vi "Autonomous Independent.vi"() -> ()   [LabVIEW 2014]
doc: "This VI is called when autonomous begins, and will automatically be terminated when autonomous ends. You can carry out timed or sensor driven robot movement independently without needing to return to the caller."
uses:
  <vilib>/Rock Robotics/WPI/Solenoid/Deprecated/WPI_SolenoidSetBool.vi
  <vilib>/Rock Robotics/Network Tables/SD Write Number.vi
  <vilib>/Rock Robotics/Network Tables/SD Read Number.vi
panel:
  out "JDF Distance":dbl
  out "JDF Speed":dbl
  out "Speed 2":dbl
  out "Speed 1":dbl
  out "Placing Distance":dbl
  out "Turning Angle":dbl
  out "Distance 2":dbl
  out "Distance 1":dbl
  in  "Reset Encoder":bool
  in  "3 Tote Data":T1
  out "Pot Value":dbl
  out "Avg Encoder":dbl
  out "R Encoder":dbl
  out "L Encoder":dbl
  # "3.5\n1.5\n80\n8\n.6\n.7"
  # "85\n4.5"
  # "Be sure to right-click and choose Data Operations>>Make Current Value default if you want to save the array values with the VI"
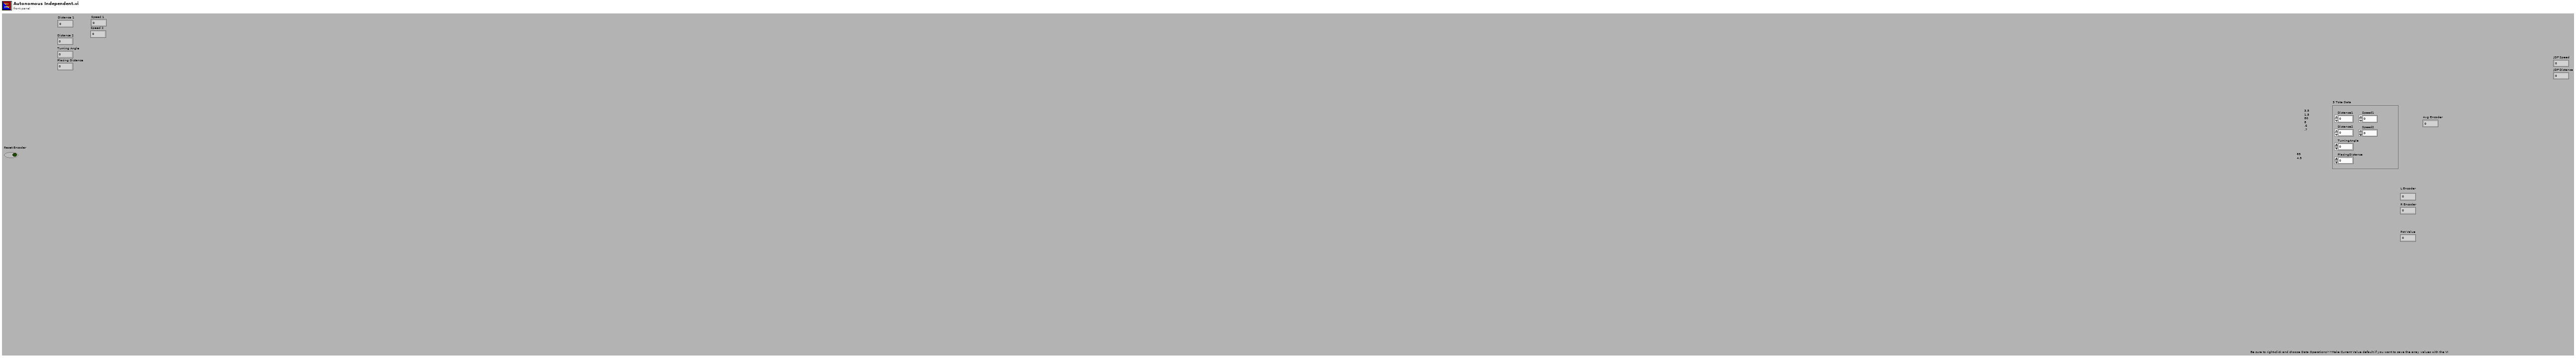
[diagram p1: front panel]
types:
  T1 = cluster{"Distance1":dbl, "Distance2":dbl, "TurningAngle":dbl, "PlacingDistance":dbl, "Speed1":dbl, "Speed2":dbl}
  T2 = typedef "WPI_SolenoidDevRef.ctl" = cluster{"DevStatus":errorcluster, "Pneumatics Control Module":u8, "Forward Solenoid Channel":T3, "Reverse Solenoid Channel":T3}
  T3 = typedef "WPI_SolenoidChannel.ctl" = enum8{"Solenoid 0", "Solenoid 1", "Solenoid 2", "Solenoid 3", "Solenoid 4", "Solenoid 5", "Solenoid 6", "Solenoid 7", "Invalid"}
  T4 = typedef "WPI_MotorControlDeviceRef.ctl" = cluster{"DeviceStatus":errorcluster, "Type":T5, "PWM":cluster{"Controller":T6, "PWM Channel":T7, "DeadBand":T8}, "CAN":cluster{"Device Number":u8, "Control Mode":T9, "Semaphore":T10, "Max Vout":dbl, "TalonSRX Control Mode":T11}, "Invert":bool, "TransformRef":T12, "InvTransformRef":T12}
  T5 = typedef "WPI_MotorControlType.ctl" = enum16{"PWM", "CAN", "CANTalonSRX"}
  T6 = typedef "FPGA_TypedefDigitalModule.ctl" = enum16{"Controller 1"}
  T7 = typedef "FPGA_DIOPWMChannel.ctl" = enum8{"PWM 0", "PWM 1", "PWM 2", "PWM 3", "PWM 4", "PWM 5", "PWM 6", "PWM 7", "PWM 8", "PWM 9", "PWM MXP 0", "PWM MXP 1", "PWM MXP 2", "PWM MXP 3", "PWM MXP 4", "PWM MXP 5", "PWM MXP 6", "PWM MXP 7", "PWM MXP 8", "PWM MXP 9", "Invalid"}
  T8 = typedef "WPI_PWMDeadband.ctl" = cluster{"Name":string, "maxPositivePwm":i32, "minPositivePwm":i32, "centerPwm":i32, "maxNegativePwm":i32, "minNegativePwm":i32, "angularRange":u16}
  T9 = typedef "WPI_CANJaguar_ControlMode.ctl" = enum8{"Percent VBus", "Current", "Speed", "Position", "Voltage"}
  T10 = typedef "Semaphore RefNum" = refnum<k1>
  T11 = typedef "WPI_CANTalonSRX_APIControlMode.ctl" = enum8{"Percent VBus", "Speed", "Position", "Slave", "Unchanged / Invalid"}
  T12 = typedef "WPI_PWMTransform_ConPane.ctl" = refnum<vi>
  T13 = typedef "WPI_RobotDriveDevRef.ctl" = cluster{"DevStatus":errorcluster, "Motors[]":T4[], "Square Inputs":bool, "Max Output":dbl}
  T14 = cluster{"SolenoidDevRef":T2, "SolenoidDevRef":T2, "MotorControlDevRef":T4, "MotorControlDevRef":T4, "SolenoidDevRef":T2, "SolenoidDevRef":T2, "SolenoidDevRef":T2}
  T15 = cluster{"SolenoidDevRef":T2, "SolenoidDevRef":T2, "MotorControlDevRef":T4, "RobotDriveDevRef":T13}
  T16 = typedef "WPI_GyroDevRef.ctl" = cluster{"DevStatus":errorcluster, "Analog Module":T17, "Analog Channel":T18, "Offset":dbl, "Gain (VoltsPerDegree/Second)":dbl}
  T17 = typedef "FPGA_TypedefAnalogModule.ctl" = enum16{"Controller 1"}
  T18 = typedef "FPGA_AIChannel.ctl" = enum8{"AI 0", "AI 1", "AI 2", "AI 3", "AI MXP 0", "AI MXP 1", "AI MXP 2", "AI MXP 3", "Invalid"}
  T19 = typedef "WPI_PotentiometerDevRef.ctl" = cluster{"DevStatus":errorcluster, "Controller":T17, "Analog Channel":T18, "Invert Output":bool}
  T20 = typedef "WPI_EncoderDevRef.ctl" = cluster{"DevStatus":errorcluster, "EncoderIndex":T21, "CounterIndex":T22, "DistancePerCount":dbl, "Decoding Type":T23}
  T21 = typedef "FPGA_EncoderIdx.ctl" = enum8{"Enc 0", "Enc 1", "Enc 2", "Enc 3", "Enc 4", "Enc 5", "Enc 6", "Enc 7", "Invalid"}
  T22 = typedef "FPGA_CounterCtrSystemIndex.ctl" = enum8{"Ctr 0", "Ctr 1", "Ctr 2", "Ctr 3", "Ctr 4", "Ctr 5", "Ctr 6", "Ctr 7", "Invalid"}
  T23 = typedef "WPI_EncoderType.ctl" = enum16{"1x", "2x", "4x"}
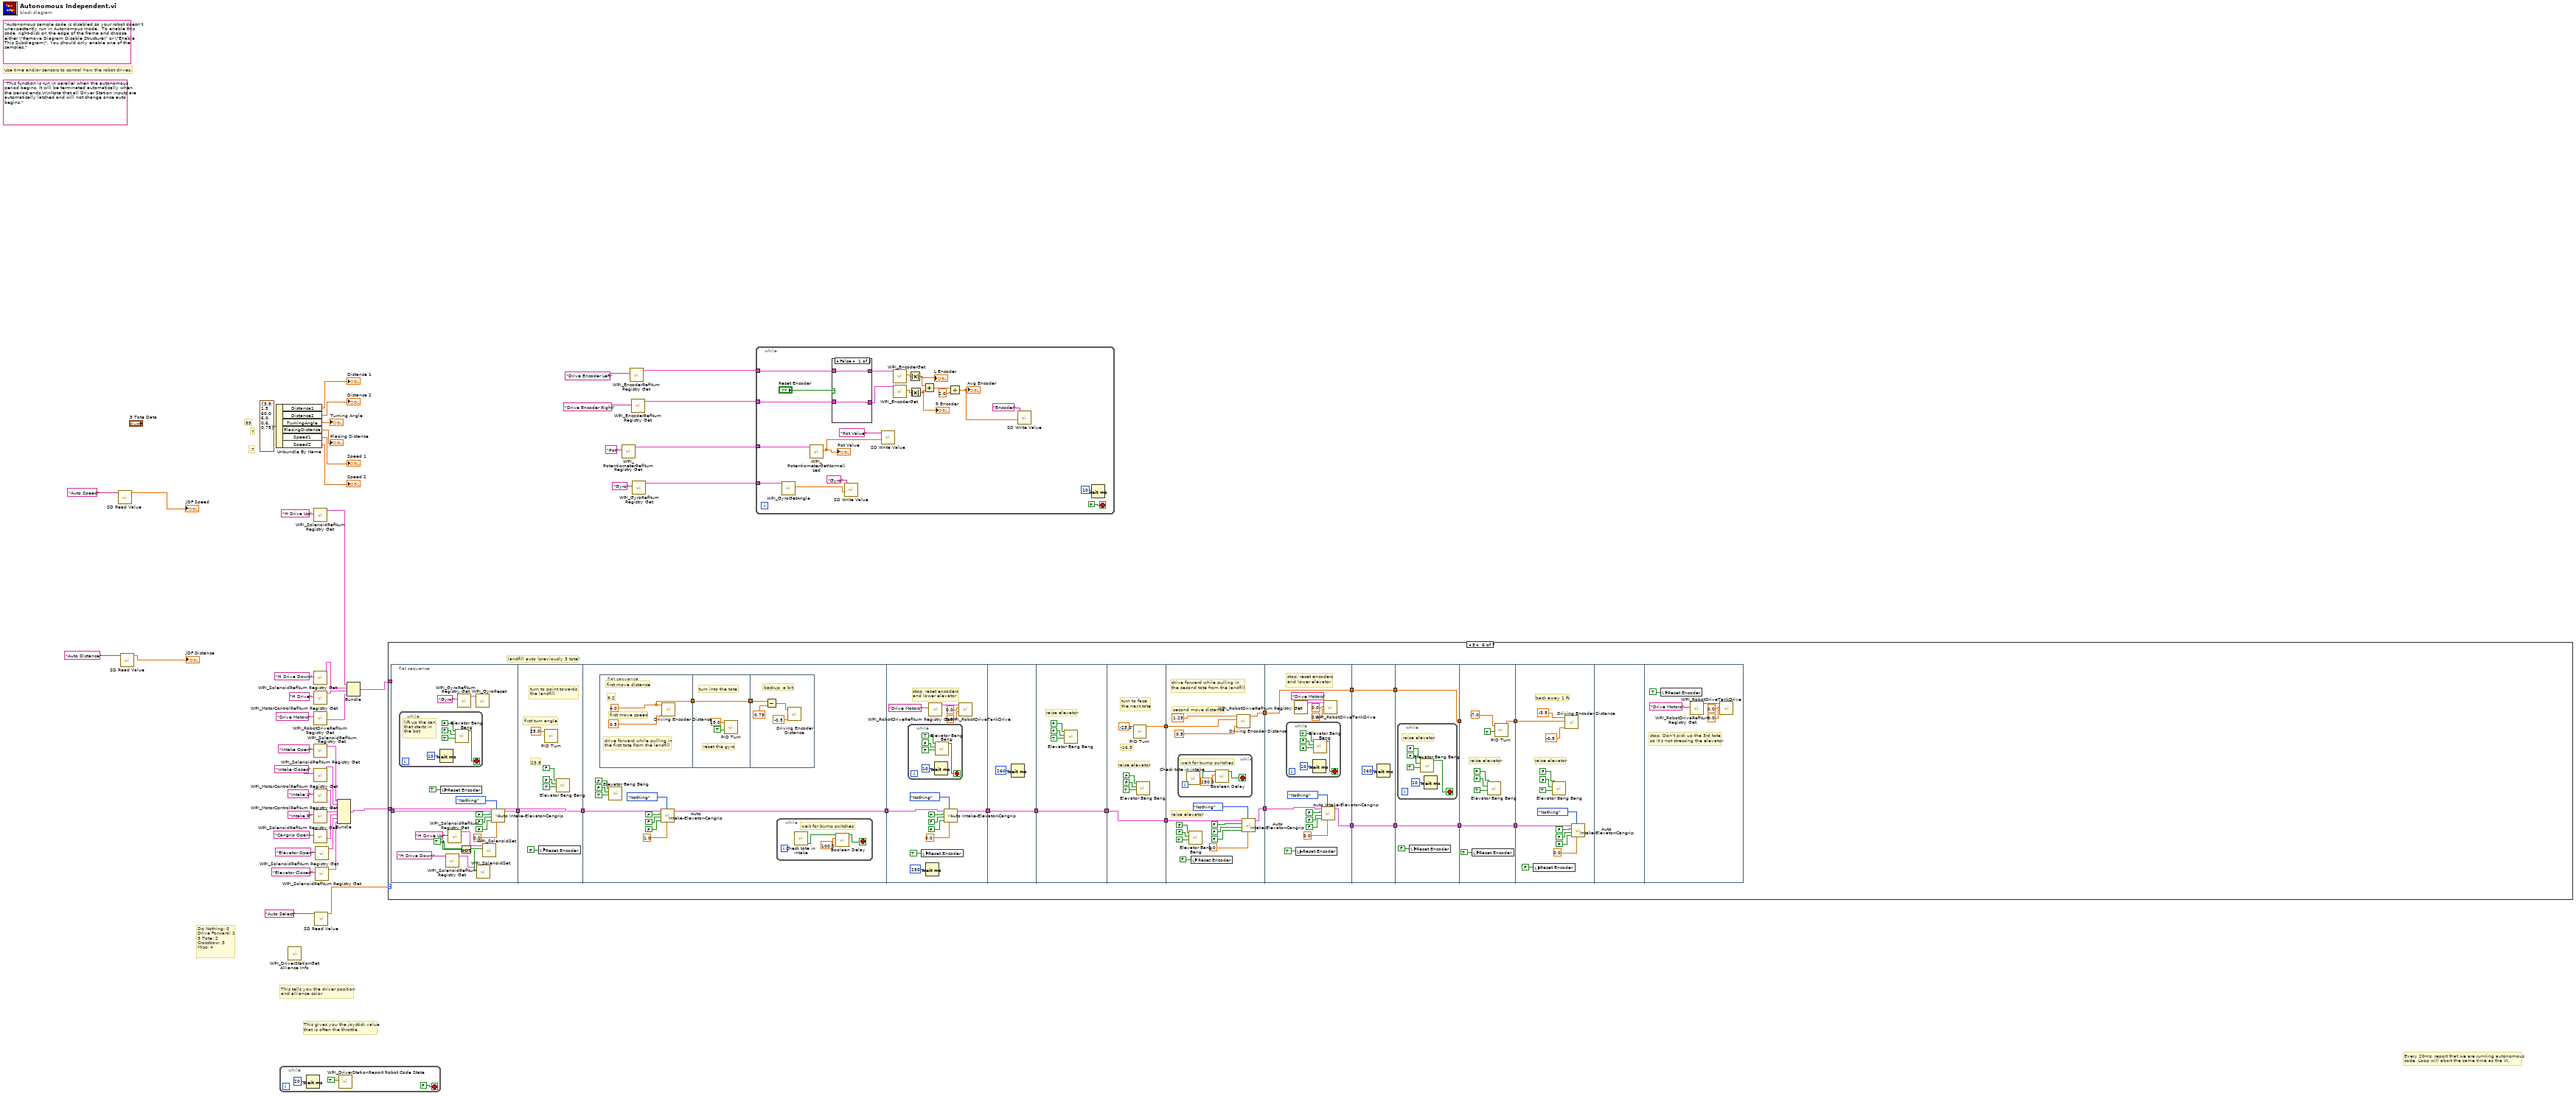
[diagram p0: block diagram]
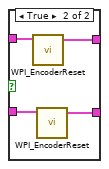
[diagram p2: hidden frame]
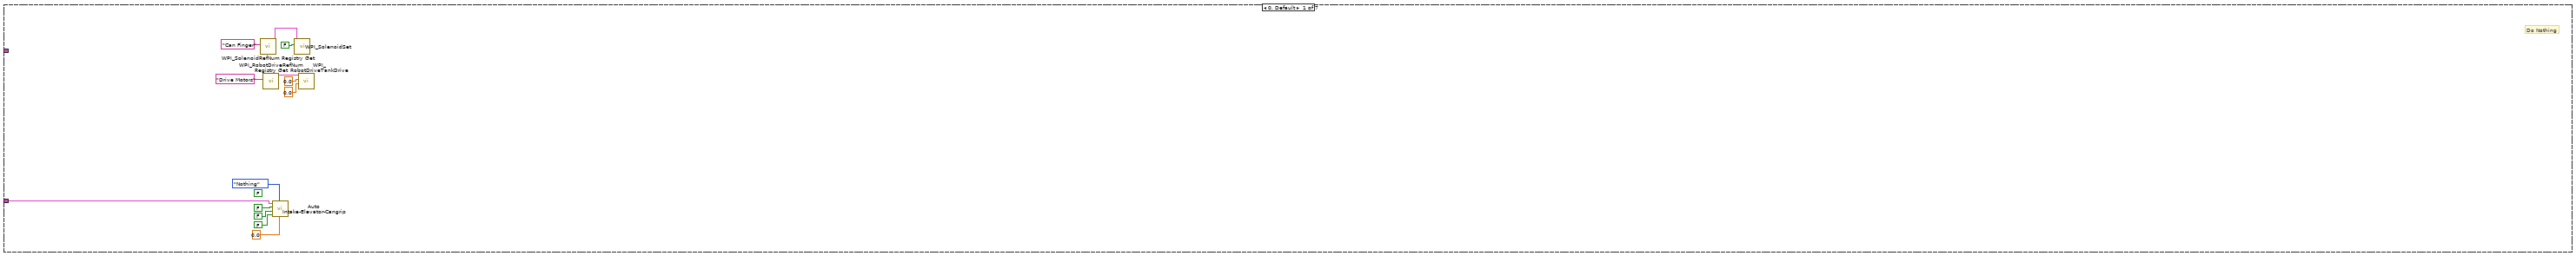
[diagram p3: hidden frame]
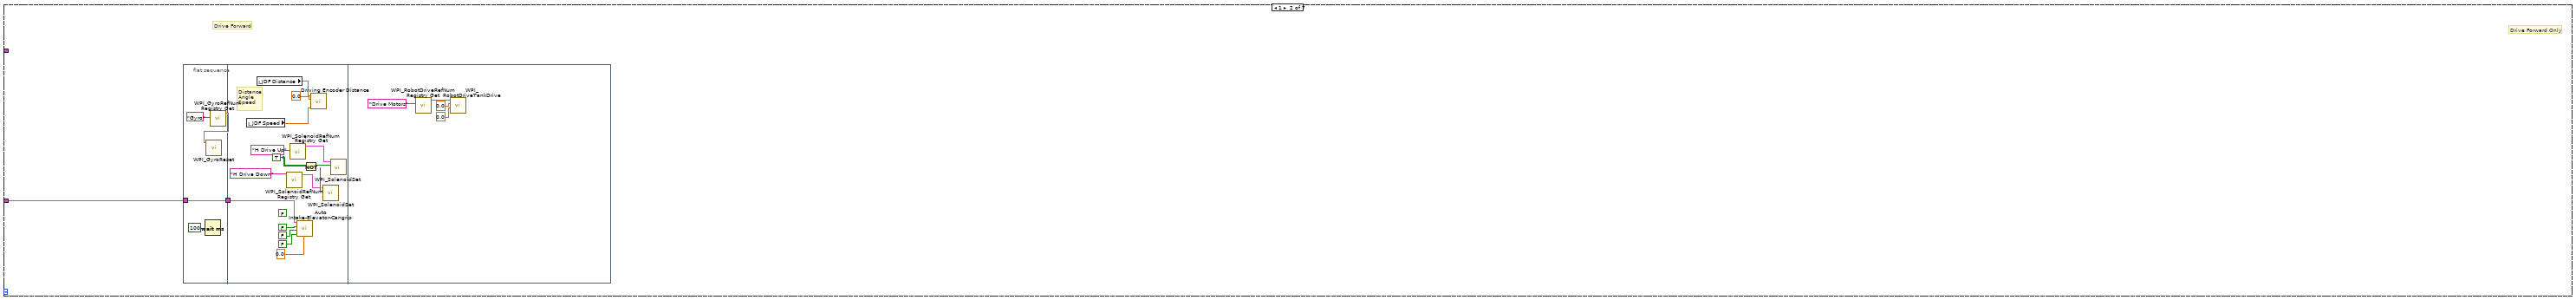
[diagram p4: hidden frame]
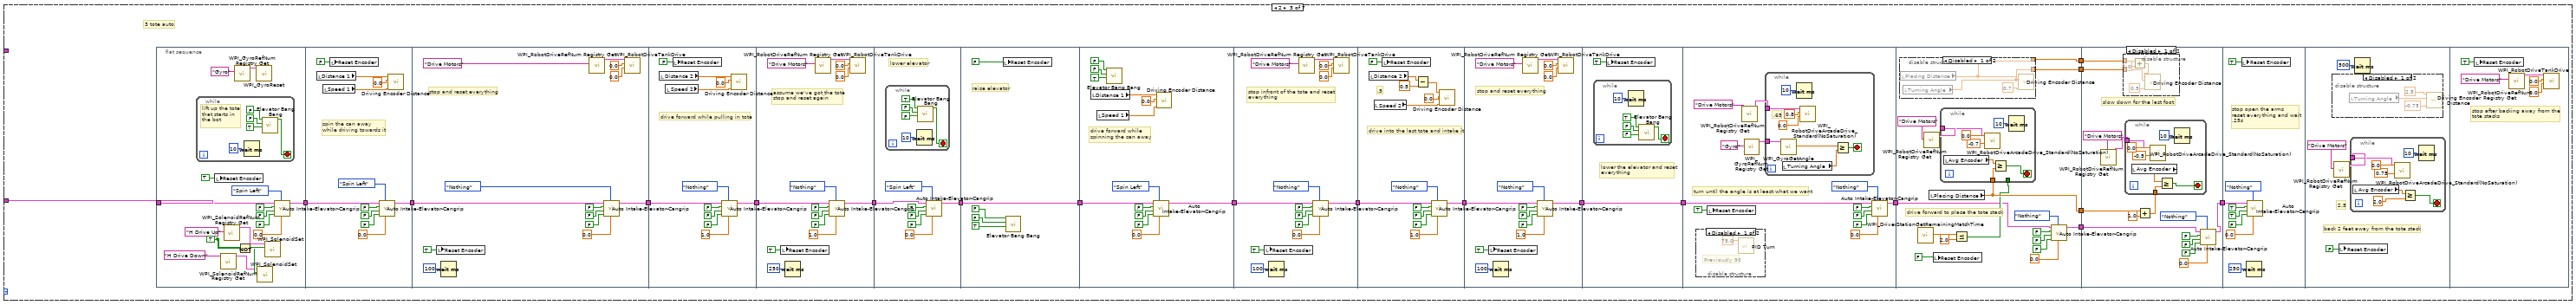
[diagram p5: hidden frame]
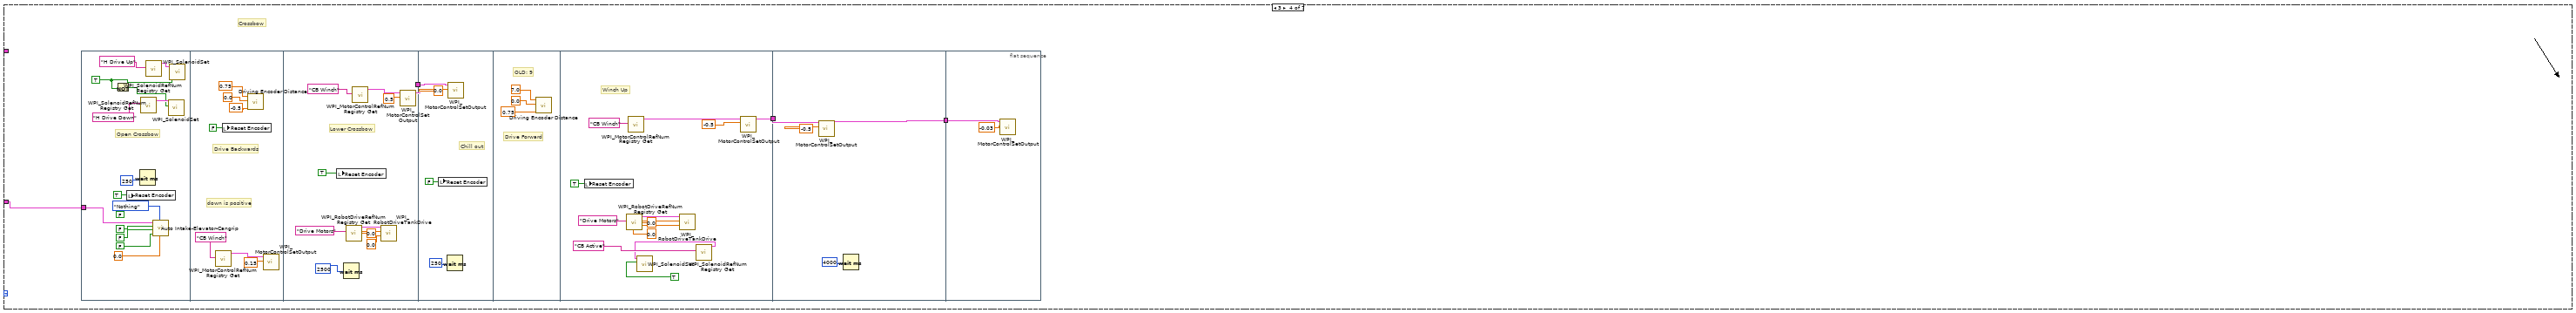
[diagram p10: hidden frame]
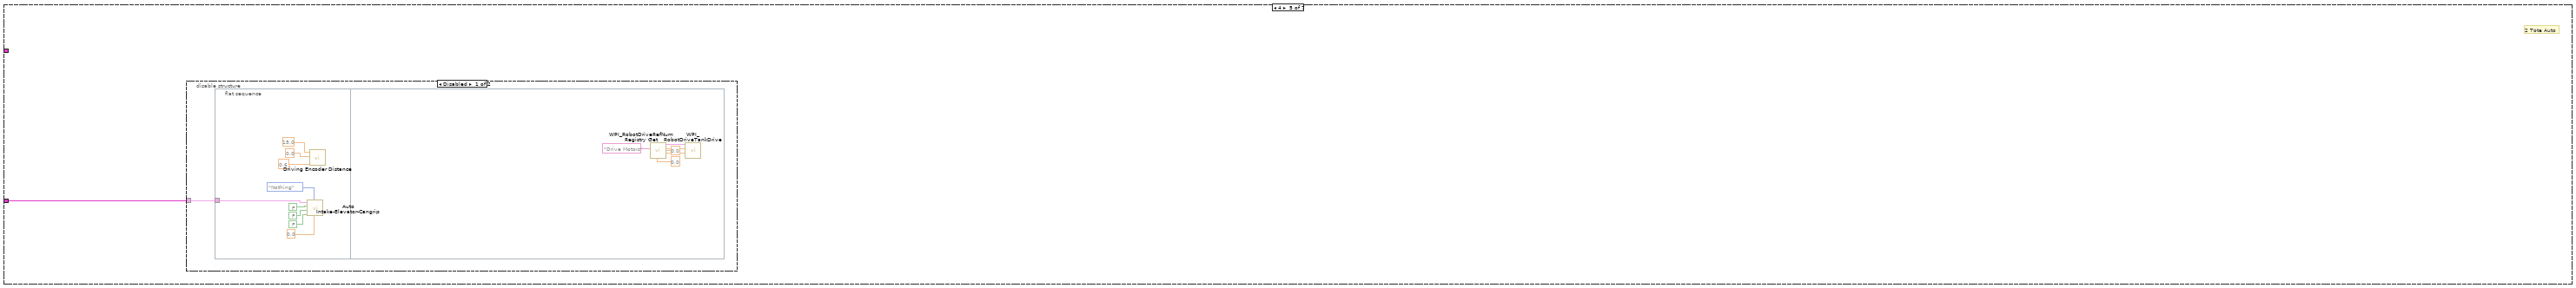
[diagram p11: hidden frame]
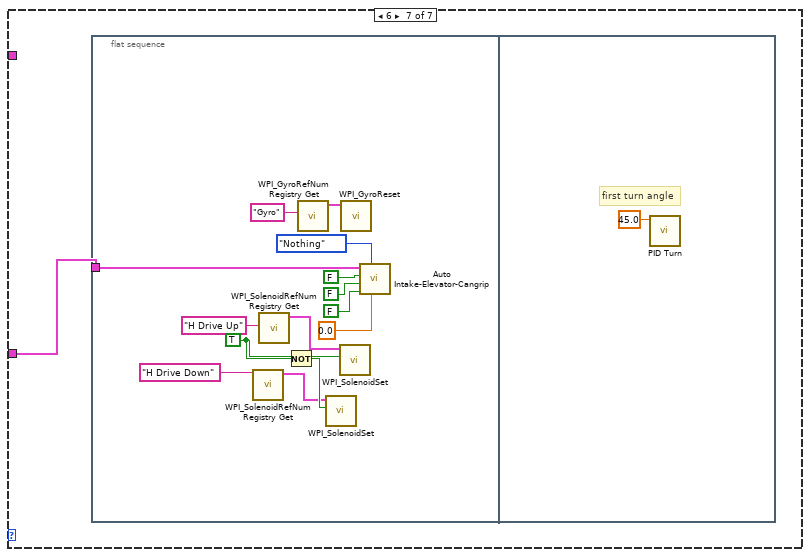
[diagram p13: hidden frame]
diagram:
  (unwired) "Autonomous sample code is disabled so your robot doesn't unexpectantly run in Autonomous mode.  To enable this code, right-click on the edge of the frame and choose either \"Remove Diagram Disable Structure\" or \"Enable This Subdiagram\". You should only enable one of the samples."
  (unwired) "This function is run in parallel when the autonomous period begins. It will be terminated automatically when the period ends.\n\nNote that all Driver Station inputs are automatically latched and will not change once auto begins."
  # "7"
  # "85"
  # ".7"
  # "Do Nothing: 0\nDrive Forward: 1\n3 Tote: 2\nCrossbow: 3\nMisc: 4"
  # "Every 20ms, report that we are running autonomous\ncode. Loop will abort the same time as the VI."
  # "This gives you the joystick value\nthat is often the throttle"
  # "Use time and/or sensors to control how the robot drives."
  # "This tells you the driver position\nand alliance color"
  n1 = call-poly <vilib>:"SD Read Value.vi"("Name"="Auto Speed") -> ("Numeric"=→"JDF Speed":dbl)  [unwired: 8 in, 2 out]
  n2 = call-poly <vilib>:"SD Read Value.vi"("Name"="Auto Distance") -> ("Numeric"=→"JDF Distance":dbl)  [unwired: 8 in, 2 out]
  n3 = Unbundle By Name(T1 {"Distance1"=3.5, "Distance2"=1.5, "TurningAngle"=60.0, "PlacingDistance"=6.0, "Speed1"=0.6, "Speed2"=0.75} ("input cluster")) -> ("Distance1"=→"Distance 1":dbl, "Distance2"=→"Distance 2":dbl, "TurningAngle"=→"Turning Angle":dbl, "PlacingDistance"=→"Placing Distance":dbl, "Speed1"=→"Speed 1":dbl, "Speed2"=→"Speed 2":dbl)
  n4 = while {
    stop <- FALSE stop-if-true
    n5 = Wait (ms)(milliseconds to wait=u32 20) -> ()  [unwired: 1 out]
    n6 = call <vilib>:"WPI_DriverStationReport Robot Code State.vi"("Autonomous"=TRUE) -> ()  [unwired: 10 in, 1 out]
  }
  n7 = call <vilib>:"WPI_DriverStationGet Alliance Info.vi"() -> ()  [unwired: 12 out]
  n8 = call <vilib>:"WPI_SolenoidRefNum Registry Get.vi"("refnum name"="H Drive Up") -> ("SolenoidDevRef"=w36:T2)  [unwired: 9 in, 1 out]
  n9 = call <vilib>:"WPI_SolenoidRefNum Registry Get.vi"("refnum name"="H Drive Down") -> ("SolenoidDevRef"=w35:T2)  [unwired: 9 in, 1 out]
  n10 = call <vilib>:"WPI_MotorControlRefNum Registry Get.vi"("refnum name"="H Drive") -> ("MotorControlDevRef"=w34:T4)  [unwired: 9 in, 1 out]
  n11 = call <vilib>:"WPI_RobotDriveRefNum Registry Get.vi"("refnum name"="Drive Motors") -> ("RobotDriveDevRef"=w33:T13)  [unwired: 1 in, 9 out]
  n12 = call <vilib>:"WPI_SolenoidRefNum Registry Get.vi"("refnum name"="Intake Open") -> ("SolenoidDevRef"=w24:T2)  [unwired: 9 in, 1 out]
  n13 = call <vilib>:"WPI_SolenoidRefNum Registry Get.vi"("refnum name"="Intake Closed") -> ("SolenoidDevRef"=w23:T2)  [unwired: 9 in, 1 out]
  n14 = call <vilib>:"WPI_MotorControlRefNum Registry Get.vi"("refnum name"="Intake L") -> ("MotorControlDevRef"=w22:T4)  [unwired: 9 in, 1 out]
  n15 = call <vilib>:"WPI_MotorControlRefNum Registry Get.vi"("refnum name"="Intake R") -> ("MotorControlDevRef"=w21:T4)  [unwired: 9 in, 1 out]
  n16 = call <vilib>:"WPI_SolenoidRefNum Registry Get.vi"("refnum name"="Cangrip Open") -> ("SolenoidDevRef"=w20:T2)  [unwired: 9 in, 1 out]
  n17 = call-poly <vilib>:"SD Read Value.vi"("Name"="Auto Select") -> ("Numeric"=w1:dbl)  [unwired: 8 in, 2 out]
  n18 = call <vilib>:"WPI_SolenoidRefNum Registry Get.vi"("refnum name"="Elevator Open") -> ("SolenoidDevRef"=w19:T2)  [unwired: 9 in, 1 out]
  n19 = call <vilib>:"WPI_SolenoidRefNum Registry Get.vi"("refnum name"="Elevator Closed") -> ("SolenoidDevRef"=w18:T2)  [unwired: 9 in, 1 out]
  n20 = Bundle("SolenoidDevRef"=w24, "SolenoidDevRef"=w23, "MotorControlDevRef"=w22, "MotorControlDevRef"=w21, "SolenoidDevRef"=w20, "SolenoidDevRef"=w19, "SolenoidDevRef"=w18) -> (w17:T14)  [unwired: 1 in]
  n21 = Bundle("SolenoidDevRef"=w36, "SolenoidDevRef"=w35, "MotorControlDevRef"=w34, "RobotDriveDevRef"=w33) -> (w32:T15)  [unwired: 1 in]
  n22 = case shown="5" w1 {
    tunnel: w32 -> [_ _ _ _ _ _ _]
    tunnel: w17 -> [w50 w63 w91 w350 w410 w443 w598]
    frame 0, Default {
      (unwired) FALSE ("Intake Spin Left")
      # "Do Nothing"
      n23 = call <vilib>:"WPI_SolenoidRefNum Registry Get.vi"("refnum name"="Can Finger") -> ("SolenoidDevRef"=w61:T2)  [unwired: 9 in, 1 out]
      n24 = call <vilib>:"WPI_RobotDriveRefNum Registry Get.vi"("refnum name"="Drive Motors") -> ("RobotDriveDevRef"=w56:T13)  [unwired: 1 in, 9 out]
      n25 = call "Auto Intake-Elevator-Cangrip.vi"("Intake Wheels (+ is in)"=0.0, "Spin Can"=enum16{"Spin Left", "Spin Right", "Nothing"}."Nothing", "Cangrip Open"=FALSE, "Elevator Open"=FALSE, "Intake Open"=FALSE, "Cluster"=w50) -> ()  [unwired: 5 in, 1 out]
      n26 = call-poly <vilib>:"WPI_SolenoidSet.vi"("Value"=FALSE, "SolenoidDevRef"=w61) -> ()  [unwired: 8 in, 2 out]
      n27 = call <vilib>:"WPI_RobotDriveTankDrive.vi"("Right axis value"=0.0, "Left axis value"=0.0, "RobotDriveDevRef"=w56) -> ()  [unwired: 6 in, 3 out]
    }
    frame 1 {
      # "Drive Forward"
      # "Drive Forward Only"
      n28 = flat-sequence {
        tunnel: w63 -> [w67]
        tunnel: [w67] -> w62
        tunnel: w62 -> [w77]
        frame #0 {
          n29 = Wait (ms)(milliseconds to wait=u32 100) -> ()  [unwired: 1 out]
          n30 = call <vilib>:"WPI_GyroRefNum Registry Get.vi"("refnum name"="Gyro") -> ("GyroDevRef"=w65:T16)  [unwired: 9 in, 1 out]
          n31 = call <vilib>:"WPI_GyroReset.vi"("GyroDevRef"=w65) -> ()  [unwired: 9 in, 2 out]
        }
        frame #1 {
          w75 = TRUE ("Reset Encoder")
          (unwired) FALSE ("Intake Spin Left")
          # "Distance\nAngle\nSpeed"
          n32 = local read "JDF Speed"() -> (w68:dbl)
          n33 = local read "JDF Distance"() -> (w69:dbl)
          n34 = call <vilib>:"WPI_SolenoidRefNum Registry Get.vi"("refnum name"="H Drive Down") -> ("SolenoidDevRef"=w73:T2)  [unwired: 9 in, 1 out]
          n35 = call <vilib>:"WPI_SolenoidRefNum Registry Get.vi"("refnum name"="H Drive Up") -> ("SolenoidDevRef"=w70:T2)  [unwired: 9 in, 1 out]
          n36 = call "Auto Intake-Elevator-Cangrip.vi"("Intake Wheels (+ is in)"=0.0, "Cangrip Open"=FALSE, "Elevator Open"=FALSE, "Intake Open"=FALSE, "Cluster"=w77) -> ()  [unwired: 6 in, 1 out]
          n37 = Not(x=w75) -> (.not. x?=w74:bool)
          n38 = call "Driving Encoder Distance.vi"("Speed"=w68, "Setpoint Angle"=0.0, "Setpoint Distance"=w69) -> ()  [unwired: 6 in, 3 out]
          n39 = call-poly <vilib>:"WPI_SolenoidSet.vi"("Value"=w74, "SolenoidDevRef"=w73) -> ()  [unwired: 8 in, 2 out]
          n40 = call-poly <vilib>:"WPI_SolenoidSet.vi"("Value"=w75, "SolenoidDevRef"=w70) -> ()  [unwired: 8 in, 2 out]
        }
        frame #2 {
          n41 = call <vilib>:"WPI_RobotDriveRefNum Registry Get.vi"("refnum name"="Drive Motors") -> ("RobotDriveDevRef"=w83:T13)  [unwired: 1 in, 9 out]
          n42 = call <vilib>:"WPI_RobotDriveTankDrive.vi"("Right axis value"=0.0, "Left axis value"=0.0, "RobotDriveDevRef"=w83) -> ()  [unwired: 6 in, 3 out]
        }
      }
    }
    frame 2 {
      # "3 tote auto"
      n43 = flat-sequence {
        tunnel: [w117] -> w104
        tunnel: w91 -> [w112]
        tunnel: [w132] -> w103
        tunnel: w104 -> [w127]
        tunnel: w103 -> [w141]
        tunnel: [w139] -> w102
        tunnel: w102 -> [w158]
        tunnel: [w154] -> w101
        tunnel: w101 -> [w169]
        tunnel: [w163] -> w100
        tunnel: [w174] -> w99
        tunnel: w100 -> [w175]
        tunnel: [w189] -> w98
        tunnel: w99 -> [w189]
        tunnel: w98 -> [w199]
        tunnel: [w198] -> w97
        tunnel: w97 -> [w207]
        tunnel: [w205] -> w96
        tunnel: w96 -> [w222]
        tunnel: [w221] -> w95
        tunnel: w95 -> [w232]
        tunnel: [w231] -> w94
        tunnel: w94 -> [w244]
        tunnel: [w244] -> w93
        tunnel: w93 -> [w257]
        tunnel: [w256] -> w92
        tunnel: w92 -> [w272]
        tunnel: [w285] -> w89
        tunnel: [w284] -> w88
        tunnel: [w281] -> w87
        tunnel: [w271] -> w86
        tunnel: [w297] -> w90
        tunnel: w89 -> [w310]
        tunnel: w88 -> [w309]
        tunnel: w87 -> [w307]
        tunnel: w86 -> [w298]
        tunnel: w90 -> [w328]
        frame #0 {
          w111 = TRUE ("Reset Encoder")
          n44 = while {
            stop <- w122 stop-if-true
            # "lift up the tote\nthat starts in \nthe bot"
            n45 = Wait (ms)(milliseconds to wait=u32 10) -> ()  [unwired: 1 out]
            n46 = call "Elevator Bang Bang.vi"("Top"=TRUE, "Middle"=FALSE, "Bottom"=FALSE) -> ("in range"=w122:bool)  [unwired: 8 in]
          }
          n47 = local write "Reset Encoder"(TRUE ("Reset Encoder")) -> ()
          n48 = call <vilib>:"WPI_SolenoidRefNum Registry Get.vi"("refnum name"="H Drive Down") -> ("SolenoidDevRef"=w107:T2)  [unwired: 9 in, 1 out]
          n49 = call <vilib>:"WPI_SolenoidRefNum Registry Get.vi"("refnum name"="H Drive Up") -> ("SolenoidDevRef"=w108:T2)  [unwired: 9 in, 1 out]
          n50 = call <vilib>:"WPI_GyroRefNum Registry Get.vi"("refnum name"="Gyro") -> ("GyroDevRef"=w119:T16)  [unwired: 9 in, 1 out]
          n51 = Not(x=w111) -> (.not. x?=w110:bool)
          n52 = call <vilib>:"WPI_GyroReset.vi"("GyroDevRef"=w119) -> ()  [unwired: 9 in, 2 out]
          n53 = call-poly <vilib>:"WPI_SolenoidSet.vi"("Value"=w110, "SolenoidDevRef"=w107) -> ()  [unwired: 8 in, 2 out]
          n54 = call-poly <vilib>:"WPI_SolenoidSet.vi"("Value"=w111, "SolenoidDevRef"=w108) -> ()  [unwired: 8 in, 2 out]
          n55 = call "Auto Intake-Elevator-Cangrip.vi"("Intake Wheels (+ is in)"=0.0, "Spin Can"=enum16{"Spin Left", "Spin Right", "Nothing"}."Spin Left", "Cangrip Open"=FALSE, "Elevator Open"=FALSE, "Intake Open"=FALSE, "Cluster"=w112) -> ("Output Cluster"=w117:T14)  [unwired: 5 in]
        }
        frame #1 {
          # "spin the can away \nwhile driving towards it"
          n56 = local read "Distance 1"() -> (w129:dbl)
          n57 = local read "Speed 1"() -> (w128:dbl)
          n58 = local write "Reset Encoder"(FALSE ("Reset Encoder")) -> ()
          n59 = call "Auto Intake-Elevator-Cangrip.vi"("Intake Wheels (+ is in)"=0.0, "Spin Can"=enum16{"Spin Left", "Spin Right", "Nothing"}."Spin Left", "Cangrip Open"=FALSE, "Elevator Open"=FALSE, "Intake Open"=FALSE, "Cluster"=w127) -> ("Output Cluster"=w132:T14)  [unwired: 5 in]
          n60 = call "Driving Encoder Distance.vi"("Speed"=w128, "Setpoint Angle"=0.0, "Setpoint Distance"=w129) -> ()  [unwired: 6 in, 3 out]
        }
        frame #2 {
          # "stop and reset everything"
          n61 = local write "Reset Encoder"(TRUE ("Reset Encoder")) -> ()
          n62 = Wait (ms)(milliseconds to wait=u32 100) -> ()  [unwired: 1 out]
          n63 = call <vilib>:"WPI_RobotDriveRefNum Registry Get.vi"("refnum name"="Drive Motors") -> ("RobotDriveDevRef"=w148:T13)  [unwired: 1 in, 9 out]
          n64 = call "Auto Intake-Elevator-Cangrip.vi"("Intake Wheels (+ is in)"=0.0, "Spin Can"=enum16{"Spin Left", "Spin Right", "Nothing"}."Nothing", "Cangrip Open"=FALSE, "Elevator Open"=FALSE, "Intake Open"=FALSE, "Cluster"=w141) -> ("Output Cluster"=w139:T14)  [unwired: 5 in]
          n65 = call <vilib>:"WPI_RobotDriveTankDrive.vi"("Right axis value"=0.0, "Left axis value"=0.0, "RobotDriveDevRef"=w148) -> ()  [unwired: 6 in, 3 out]
        }
        frame #3 {
          # "drive forward while pulling in tote"
          n66 = local read "Distance 2"() -> (w152:dbl)
          n67 = local read "Speed 2"() -> (w151:dbl)
          n68 = local write "Reset Encoder"(FALSE ("Reset Encoder")) -> ()
          n69 = call "Auto Intake-Elevator-Cangrip.vi"("Intake Wheels (+ is in)"=1.0, "Spin Can"=enum16{"Spin Left", "Spin Right", "Nothing"}."Nothing", "Cangrip Open"=FALSE, "Elevator Open"=FALSE, "Intake Open"=FALSE, "Cluster"=w158) -> ("Output Cluster"=w154:T14)  [unwired: 5 in]
          n70 = call "Driving Encoder Distance.vi"("Speed"=w151, "Setpoint Angle"=0.0, "Setpoint Distance"=w152) -> ()  [unwired: 6 in, 3 out]
        }
        frame #4 {
          # "assume we've got the tote\nstop and reset again"
          n71 = local write "Reset Encoder"(TRUE ("Reset Encoder")) -> ()
          n72 = Wait (ms)(milliseconds to wait=u32 250) -> ()  [unwired: 1 out]
          n73 = call <vilib>:"WPI_RobotDriveRefNum Registry Get.vi"("refnum name"="Drive Motors") -> ("RobotDriveDevRef"=w166:T13)  [unwired: 1 in, 9 out]
          n74 = call "Auto Intake-Elevator-Cangrip.vi"("Intake Wheels (+ is in)"=1.0, "Spin Can"=enum16{"Spin Left", "Spin Right", "Nothing"}."Nothing", "Cangrip Open"=FALSE, "Elevator Open"=FALSE, "Intake Open"=FALSE, "Cluster"=w169) -> ("Output Cluster"=w163:T14)  [unwired: 5 in]
          n75 = call <vilib>:"WPI_RobotDriveTankDrive.vi"("Right axis value"=0.0, "Left axis value"=0.0, "RobotDriveDevRef"=w166) -> ()  [unwired: 6 in, 3 out]
        }
        frame #5 {
          # "lower elevator"
          n76 = while {
            stop <- w182 stop-if-true
            n77 = Wait (ms)(milliseconds to wait=u32 10) -> ()  [unwired: 1 out]
            n78 = call "Elevator Bang Bang.vi"("Top"=FALSE, "Middle"=FALSE, "Bottom"=TRUE) -> ("in range"=w182:bool)  [unwired: 8 in]
          }
          n79 = call "Auto Intake-Elevator-Cangrip.vi"("Intake Wheels (+ is in)"=0.0, "Spin Can"=enum16{"Spin Left", "Spin Right", "Nothing"}."Spin Left", "Cangrip Open"=FALSE, "Elevator Open"=FALSE, "Intake Open"=FALSE, "Cluster"=w175) -> ("Output Cluster"=w174:T14)  [unwired: 5 in]
        }
        frame #6 {
          # "raise elevator"
          n80 = local write "Reset Encoder"(FALSE ("Reset Encoder")) -> ()
          n81 = call "Elevator Bang Bang.vi"("Top"=TRUE, "Middle"=FALSE, "Bottom"=FALSE) -> ()  [unwired: 8 in, 1 out]
        }
        frame #7 {
          # "drive forward while \nspinning the can away"
          n82 = local read "Distance 1"() -> (w193:dbl)
          n83 = local read "Speed 1"() -> (w194:dbl)
          n84 = call "Elevator Bang Bang.vi"("Top"=TRUE, "Middle"=FALSE, "Bottom"=FALSE) -> ()  [unwired: 8 in, 1 out]
          n85 = call "Auto Intake-Elevator-Cangrip.vi"("Intake Wheels (+ is in)"=0.0, "Spin Can"=enum16{"Spin Left", "Spin Right", "Nothing"}."Spin Left", "Cangrip Open"=FALSE, "Elevator Open"=FALSE, "Intake Open"=FALSE, "Cluster"=w199) -> ("Output Cluster"=w198:T14)  [unwired: 5 in]
          n86 = call "Driving Encoder Distance.vi"("Speed"=w194, "Setpoint Angle"=0.0, "Setpoint Distance"=w193) -> ()  [unwired: 6 in, 3 out]
        }
        frame #8 {
          # "stop infront of the tote and reset\neverything"
          n87 = local write "Reset Encoder"(TRUE ("Reset Encoder")) -> ()
          n88 = Wait (ms)(milliseconds to wait=u32 100) -> ()  [unwired: 1 out]
          n89 = call <vilib>:"WPI_RobotDriveRefNum Registry Get.vi"("refnum name"="Drive Motors") -> ("RobotDriveDevRef"=w214:T13)  [unwired: 1 in, 9 out]
          n90 = call "Auto Intake-Elevator-Cangrip.vi"("Intake Wheels (+ is in)"=0.0, "Spin Can"=enum16{"Spin Left", "Spin Right", "Nothing"}."Nothing", "Cangrip Open"=FALSE, "Elevator Open"=FALSE, "Intake Open"=FALSE, "Cluster"=w207) -> ("Output Cluster"=w205:T14)  [unwired: 5 in]
          n91 = call <vilib>:"WPI_RobotDriveTankDrive.vi"("Right axis value"=0.0, "Left axis value"=0.0, "RobotDriveDevRef"=w214) -> ()  [unwired: 6 in, 3 out]
        }
        frame #9 {
          # "drive into the last tote and intake it"
          # ".5"
          n92 = local read "Distance 2"() -> (w220:dbl)
          n93 = local read "Speed 2"() -> (w229:dbl)
          n94 = local write "Reset Encoder"(FALSE ("Reset Encoder")) -> ()
          n95 = Subtract(x=w220, y=0.5) -> (x-y=w219:dbl)
          n96 = call "Auto Intake-Elevator-Cangrip.vi"("Intake Wheels (+ is in)"=1.0, "Spin Can"=enum16{"Spin Left", "Spin Right", "Nothing"}."Nothing", "Cangrip Open"=FALSE, "Elevator Open"=FALSE, "Intake Open"=FALSE, "Cluster"=w222) -> ("Output Cluster"=w221:T14)  [unwired: 5 in]
          n97 = call "Driving Encoder Distance.vi"("Speed"=w229, "Setpoint Angle"=0.0, "Setpoint Distance"=w219) -> ()  [unwired: 6 in, 3 out]
        }
        frame #10 {
          # "stop and reset everything"
          n98 = local write "Reset Encoder"(TRUE ("Reset Encoder")) -> ()
          n99 = Wait (ms)(milliseconds to wait=u32 100) -> ()  [unwired: 1 out]
          n100 = call <vilib>:"WPI_RobotDriveRefNum Registry Get.vi"("refnum name"="Drive Motors") -> ("RobotDriveDevRef"=w239:T13)  [unwired: 1 in, 9 out]
          n101 = call "Auto Intake-Elevator-Cangrip.vi"("Intake Wheels (+ is in)"=1.0, "Spin Can"=enum16{"Spin Left", "Spin Right", "Nothing"}."Nothing", "Cangrip Open"=FALSE, "Elevator Open"=FALSE, "Intake Open"=FALSE, "Cluster"=w232) -> ("Output Cluster"=w231:T14)  [unwired: 5 in]
          n102 = call <vilib>:"WPI_RobotDriveTankDrive.vi"("Right axis value"=0.0, "Left axis value"=0.0, "RobotDriveDevRef"=w239) -> ()  [unwired: 6 in, 3 out]
        }
        frame #11 {
          # "lower the elevator and reset\neverything"
          n103 = while {
            stop <- w246 stop-if-true
            n104 = Wait (ms)(milliseconds to wait=u32 10) -> ()  [unwired: 1 out]
            n105 = call "Elevator Bang Bang.vi"("Top"=FALSE, "Middle"=FALSE, "Bottom"=TRUE) -> ("in range"=w246:bool)  [unwired: 8 in]
          }
          n106 = local write "Reset Encoder"(TRUE ("Reset Encoder")) -> ()
        }
        frame #12 {
          # "turn until the angle is at least what we want"
          n107 = disable-structure shown="Disabled" {
            frame Disabled {
              # "Previously 90"
              n108 = call "PID Turn.vi"("Setpoint"=75.0) -> ()  [unwired: 10 in, 1 out]
            }
            frame Enabled {
            }
          }
          n109 = local write "Reset Encoder"(TRUE ("Reset Encoder")) -> ()
          n110 = call <vilib>:"WPI_RobotDriveRefNum Registry Get.vi"("refnum name"="Drive Motors") -> ("RobotDriveDevRef"=w251:T13)  [unwired: 1 in, 9 out]
          n111 = call <vilib>:"WPI_GyroRefNum Registry Get.vi"("refnum name"="Gyro") -> ("GyroDevRef"=w252:T16)  [unwired: 9 in, 1 out]
          n112 = while {
            tunnel: w252 -> [w268]
            tunnel: w251 -> [w266]
            stop <- w269 stop-if-true
            # ".65"
            n113 = call <vilib>:"WPI_GyroGetAngle.vi"("GyroDevRef"=w268) -> ("Angle"=w270:dbl)  [unwired: 7 in, 3 out]
            n114 = local read "Turning Angle"() -> (w263:dbl)
            n115 = Wait (ms)(milliseconds to wait=u32 10) -> ()  [unwired: 1 out]
            n116 = call <vilib>:"WPI_RobotDriveArcadeDrive_Standard(NoSaturation).vi"("Y axis value"=0.0, "X axis value"=0.8, "RobotDriveDevRef"=w266) -> ()  [unwired: 1 in, 8 out]
            n117 = Greater Or Equal?(x=w270, y=w263) -> (x >= y?=w269:bool)
          }
          n118 = call "Auto Intake-Elevator-Cangrip.vi"("Intake Wheels (+ is in)"=0.0, "Spin Can"=enum16{"Spin Left", "Spin Right", "Nothing"}."Nothing", "Cangrip Open"=FALSE, "Elevator Open"=FALSE, "Intake Open"=FALSE, "Cluster"=w257) -> ("Output Cluster"=w256:T14)  [unwired: 5 in]
        }
        frame #13 {
          # "drive forward to place the tote stack"
          n119 = disable-structure shown="Disabled" {
            disable-tunnel: [w288 _] -> w285
            disable-tunnel: [w287 _] -> w284
            frame Disabled {
              n120 = local read "Placing Distance"() -> (w287:dbl)
              n121 = local read "Turning Angle"() -> (w288:dbl)
              n122 = call "Driving Encoder Distance.vi"("Speed"=0.7, "Setpoint Angle"=w288, "Setpoint Distance"=w287) -> ()  [unwired: 6 in, 3 out]
            }
            frame Enabled {
            }
          }
          n123 = call <vilib>:"WPI_DriverStationGetRemainingMatchTime.vi"() -> ("Match Time(s)"=w280:sgl)  [unwired: 10 in, 1 out]
          n124 = call <vilib>:"WPI_RobotDriveRefNum Registry Get.vi"("refnum name"="Drive Motors") -> ("RobotDriveDevRef"=w283:T13)  [unwired: 9 in, 1 out]
          n125 = local read "Placing Distance"() -> (w281:dbl)
          n126 = local write "Reset Encoder"(FALSE ("Reset Encoder")) -> ()
          n127 = Less Or Equal?(x=w280, y=sgl 2.0) -> (x <= y?=w278:bool)
          n128 = while {
            tunnel: w283 -> [w294]
            tunnel: w281 -> [w292]
            tunnel: w278 -> [_]
            stop <- w290 stop-if-true
            n129 = local read "Avg Encoder"() -> (w291:dbl)
            n130 = call <vilib>:"WPI_RobotDriveArcadeDrive_Standard(NoSaturation).vi"("Y axis value"=-0.7, "X axis value"=0.0, "RobotDriveDevRef"=w294) -> ()  [unwired: 1 in, 8 out]
            n131 = Greater Or Equal?(x=w291, y=w292) -> (x >= y?=w290:bool)
            n132 = Wait (ms)(milliseconds to wait=u32 10) -> ()  [unwired: 1 out]
          }
          n133 = call "Auto Intake-Elevator-Cangrip.vi"("Intake Wheels (+ is in)"=0.0, "Spin Can"=enum16{"Spin Left", "Spin Right", "Nothing"}."Nothing", "Cangrip Open"=FALSE, "Elevator Open"=FALSE, "Intake Open"=FALSE, "Cluster"=w272) -> ("Output Cluster"=w271:T14)  [unwired: 5 in]
        }
        frame #14 {
          # "slow down for the last foot"
          n134 = call <vilib>:"WPI_RobotDriveRefNum Registry Get.vi"("refnum name"="Drive Motors") -> ("RobotDriveDevRef"=w304:T13)  [unwired: 9 in, 1 out]
          n135 = disable-structure shown="Disabled" {
            disable-tunnel: w310 -> [w314 _]
            disable-tunnel: w309 -> [w312 _]
            frame Disabled {
              n136 = Add(x=w312, y=1.0) -> (x+y=w311:dbl)
              n137 = call "Driving Encoder Distance.vi"("Speed"=0.5, "Setpoint Angle"=w314, "Setpoint Distance"=w311) -> ()  [unwired: 6 in, 3 out]
            }
            frame Enabled {
            }
          }
          n138 = Add(x=w307, y=1.0) -> (x+y=w308:dbl)
          n139 = while {
            tunnel: w308 -> [w319]
            tunnel: w304 -> [w317]
            stop <- w316 stop-if-true
            n140 = local read "Avg Encoder"() -> (w318:dbl)
            n141 = call <vilib>:"WPI_RobotDriveArcadeDrive_Standard(NoSaturation).vi"("Y axis value"=-0.5, "X axis value"=0.0, "RobotDriveDevRef"=w317) -> ()  [unwired: 1 in, 8 out]
            n142 = Greater Or Equal?(x=w318, y=w319) -> (x >= y?=w316:bool)
            n143 = Wait (ms)(milliseconds to wait=u32 10) -> ()  [unwired: 1 out]
          }
          n144 = call "Auto Intake-Elevator-Cangrip.vi"("Intake Wheels (+ is in)"=0.0, "Spin Can"=enum16{"Spin Left", "Spin Right", "Nothing"}."Nothing", "Cangrip Open"=FALSE, "Elevator Open"=FALSE, "Intake Open"=FALSE, "Cluster"=w298) -> ("Output Cluster"=w297:T14)  [unwired: 5 in]
        }
        frame #15 {
          # "stop open the arms\nreset everything and wait\n.25s"
          n145 = local write "Reset Encoder"(TRUE) -> ()
          n146 = Wait (ms)(milliseconds to wait=u32 250) -> ()  [unwired: 1 out]
          n147 = call "Auto Intake-Elevator-Cangrip.vi"("Intake Wheels (+ is in)"=0.0, "Spin Can"=enum16{"Spin Left", "Spin Right", "Nothing"}."Nothing", "Cangrip Open"=FALSE, "Elevator Open"=TRUE, "Intake Open"=TRUE, "Cluster"=w328) -> ()  [unwired: 5 in, 1 out]
        }
        frame #16 {
          # "back 2 feet away from the tote stack"
          # "2.5"
          n148 = disable-structure shown="Disabled" {
            frame Disabled {
              n149 = local read "Turning Angle"() -> (w336:dbl)
              n150 = call "Driving Encoder Distance.vi"("Speed"=-0.75, "Setpoint Angle"=w336, "Setpoint Distance"=2.5) -> ()  [unwired: 6 in, 3 out]
            }
            frame Enabled {
            }
          }
          n151 = call <vilib>:"WPI_RobotDriveRefNum Registry Get.vi"("refnum name"="Drive Motors") -> ("RobotDriveDevRef"=w331:T13)  [unwired: 9 in, 1 out]
          n152 = local write "Reset Encoder"(FALSE ("Reset Encoder")) -> ()
          n153 = while {
            tunnel: w331 -> [w342]
            stop <- w340 stop-if-true
            n154 = local read "Avg Encoder"() -> (w339:dbl)
            n155 = call <vilib>:"WPI_RobotDriveArcadeDrive_Standard(NoSaturation).vi"("Y axis value"=0.75, "X axis value"=0.0, "RobotDriveDevRef"=w342) -> ()  [unwired: 1 in, 8 out]
            n156 = Greater Or Equal?(x=w339, y=2.0 ("Placing Distance")) -> (x >= y?=w340:bool)
            n157 = Wait (ms)(milliseconds to wait=u32 10) -> ()  [unwired: 1 out]
          }
          n158 = Wait (ms)(milliseconds to wait=u32 500) -> ()  [unwired: 1 out]
        }
        frame #17 {
          # "stop after backing away from the\ntote stacks"
          n159 = local write "Reset Encoder"(TRUE ("Reset Encoder")) -> ()
          n160 = call <vilib>:"WPI_RobotDriveRefNum Registry Get.vi"("refnum name"="Drive Motors") -> ("RobotDriveDevRef"=w348:T13)  [unwired: 1 in, 9 out]
          n161 = call <vilib>:"WPI_RobotDriveTankDrive.vi"("Right axis value"=0.0, "Left axis value"=0.0, "RobotDriveDevRef"=w348) -> ()  [unwired: 6 in, 3 out]
        }
      }
    }
    frame 3 {
      # "Crossbow"
      n162 = flat-sequence {
        tunnel: w350 -> [w355]
        tunnel: [w375] -> w353
        tunnel: w353 -> [w388]
        tunnel: [w396] -> w352
        tunnel: w352 -> [w406]
        tunnel: [w404] -> w351
        tunnel: w351 -> [w408]
        frame #0 {
          w359 = TRUE ("Reset Encoder")
          (unwired) FALSE ("Intake Spin Left")
          # "Open Crossbow"
          n163 = Not(x=w359) -> (.not. x?=w360:bool)
          n164 = local write "Reset Encoder"(TRUE ("Reset Encoder")) -> ()
          n165 = Wait (ms)(milliseconds to wait=u32 250) -> ()  [unwired: 1 out]
          n166 = call <vilib>:"WPI_SolenoidRefNum Registry Get.vi"("refnum name"="H Drive Down") -> ("SolenoidDevRef"=w362:T2)  [unwired: 9 in, 1 out]
          n167 = call <vilib>:"WPI_SolenoidRefNum Registry Get.vi"("refnum name"="H Drive Up") -> ("SolenoidDevRef"=w363:T2)  [unwired: 9 in, 1 out]
          n168 = call "Auto Intake-Elevator-Cangrip.vi"("Intake Wheels (+ is in)"=0.0, "Spin Can"=enum16{"Spin Left", "Spin Right", "Nothing"}."Nothing", "Cangrip Open"=FALSE, "Elevator Open"=FALSE, "Intake Open"=FALSE, "Cluster"=w355) -> ()  [unwired: 5 in, 1 out]
          n169 = call-poly <vilib>:"WPI_SolenoidSet.vi"("Value"=w360, "SolenoidDevRef"=w362) -> ()  [unwired: 8 in, 2 out]
          n170 = call-poly <vilib>:"WPI_SolenoidSet.vi"("Value"=w359, "SolenoidDevRef"=w363) -> ()  [unwired: 8 in, 2 out]
        }
        frame #1 {
          # "down is positive"
          # "Drive Backwards"
          n171 = call <vilib>:"WPI_MotorControlRefNum Registry Get.vi"("refnum name"="CB Winch") -> ("MotorControlDevRef"=w370:T4)  [unwired: 9 in, 1 out]
          n172 = local write "Reset Encoder"(FALSE ("Reset Encoder")) -> ()
          n173 = call "Driving Encoder Distance.vi"("Speed"=-0.5, "Setpoint Angle"=0.0, "Setpoint Distance"=0.75) -> ()  [unwired: 6 in, 3 out]
          n174 = call <vilib>:"WPI_MotorControlSetOutput.vi"("Output"=0.15, "MotorControlDevRef"=w370) -> ()  [unwired: 7 in, 3 out]
        }
        frame #2 {
          # "Lower Crossbow"
          n175 = local write "Reset Encoder"(TRUE ("Reset Encoder")) -> ()
          n176 = Wait (ms)(milliseconds to wait=u32 2500) -> ()  [unwired: 1 out]
          n177 = call <vilib>:"WPI_RobotDriveRefNum Registry Get.vi"("refnum name"="Drive Motors") -> ("RobotDriveDevRef"=w376:T13)  [unwired: 1 in, 9 out]
          n178 = call <vilib>:"WPI_MotorControlRefNum Registry Get.vi"("refnum name"="CB Winch") -> ("MotorControlDevRef"=w384:T4)  [unwired: 9 in, 1 out]
          n179 = call <vilib>:"WPI_RobotDriveTankDrive.vi"("Right axis value"=0.0, "Left axis value"=0.0, "RobotDriveDevRef"=w376) -> ()  [unwired: 6 in, 3 out]
          n180 = call <vilib>:"WPI_MotorControlSetOutput.vi"("Output"=0.5, "MotorControlDevRef"=w384) -> ("MotorControlDevRef"=w375:T4)  [unwired: 7 in, 2 out]
        }
        frame #3 {
          # "Chill out"
          n181 = local write "Reset Encoder"(FALSE ("Reset Encoder")) -> ()
          n182 = Wait (ms)(milliseconds to wait=u32 250) -> ()  [unwired: 1 out]
          n183 = call <vilib>:"WPI_MotorControlSetOutput.vi"("Output"=0.0, "MotorControlDevRef"=w388) -> ()  [unwired: 7 in, 3 out]
        }
        frame #4 {
          # "OLD: 9"
          # "Drive Forward"
          n184 = call "Driving Encoder Distance.vi"("Speed"=0.75, "Setpoint Angle"=0.0, "Setpoint Distance"=7.0) -> ()  [unwired: 6 in, 3 out]
        }
        frame #5 {
          # "Winch Up"
          n185 = local write "Reset Encoder"(TRUE ("Reset Encoder")) -> ()
          n186 = call <vilib>:"WPI_RobotDriveRefNum Registry Get.vi"("refnum name"="Drive Motors") -> ("RobotDriveDevRef"=w401:T13)  [unwired: 1 in, 9 out]
          n187 = call <vilib>:"WPI_MotorControlRefNum Registry Get.vi"("refnum name"="CB Winch") -> ("MotorControlDevRef"=w403:T4)  [unwired: 9 in, 1 out]
          n188 = call <vilib>:"WPI_RobotDriveTankDrive.vi"("Right axis value"=0.0, "Left axis value"=0.0, "RobotDriveDevRef"=w401) -> ()  [unwired: 6 in, 3 out]
          n189 = call <vilib>:"WPI_SolenoidRefNum Registry Get.vi"("refnum name"="CB Active") -> ("SolenoidDevRef"=w392:T2)  [unwired: 9 in, 1 out]
          n190 = call-poly <vilib>:"WPI_SolenoidSet.vi"("Value"=TRUE ("Button Intake Open"), "SolenoidDevRef"=w392) -> ()  [unwired: 8 in, 2 out]
          n191 = call <vilib>:"WPI_MotorControlSetOutput.vi"("Output"=-0.5, "MotorControlDevRef"=w403) -> ("MotorControlDevRef"=w396:T4)  [unwired: 7 in, 2 out]
        }
        frame #6 {
          n192 = call <vilib>:"WPI_MotorControlSetOutput.vi"("Output"=-0.5, "MotorControlDevRef"=w406) -> ("MotorControlDevRef"=w404:T4)  [unwired: 7 in, 2 out]
          n193 = Wait (ms)(milliseconds to wait=u32 4000) -> ()  [unwired: 1 out]
        }
        frame #7 {
          n194 = call <vilib>:"WPI_MotorControlSetOutput.vi"("Output"=-0.03, "MotorControlDevRef"=w408) -> ()  [unwired: 7 in, 3 out]
        }
      }
    }
    frame 4 {
      # "2 Tote Auto"
      n195 = disable-structure shown="Disabled" {
        disable-tunnel: w410 -> [w411 _]
        frame Disabled {
          n196 = flat-sequence {
            tunnel: w411 -> [w412]
            frame #0 {
              n197 = call "Auto Intake-Elevator-Cangrip.vi"("Intake Wheels (+ is in)"=0.0, "Spin Can"=enum16{"Spin Left", "Spin Right", "Nothing"}."Nothing", "Cangrip Open"=FALSE, "Elevator Open"=FALSE, "Intake Open"=FALSE, "Cluster"=w412) -> ()  [unwired: 5 in, 1 out]
              n198 = call "Driving Encoder Distance.vi"("Speed"=0.6, "Setpoint Angle"=0.0, "Setpoint Distance"=15.0) -> ()  [unwired: 6 in, 3 out]
            }
            frame #1 {
              n199 = call <vilib>:"WPI_RobotDriveRefNum Registry Get.vi"("refnum name"="Drive Motors") -> ("RobotDriveDevRef"=w424:T13)  [unwired: 1 in, 9 out]
              n200 = call <vilib>:"WPI_RobotDriveTankDrive.vi"("Right axis value"=0.0, "Left axis value"=0.0, "RobotDriveDevRef"=w424) -> ()  [unwired: 6 in, 3 out]
            }
          }
        }
        frame Enabled {
        }
      }
    }
    frame 5 {
      # "landfill auto (previously 3 tote)"
      n201 = flat-sequence {
        tunnel: w443 -> [w452]
        tunnel: [w444] -> w442
        tunnel: w442 -> [w470]
        tunnel: [w470] -> w441
        tunnel: w441 -> [w477]
        tunnel: [w476] -> w437
        tunnel: [w502] -> w434
        tunnel: w437 -> [w495]
        tunnel: w434 -> [w514]
        tunnel: [w514] -> w433
        tunnel: w433 -> [w515]
        tunnel: [w515] -> w438
        tunnel: [w523] -> w440
        tunnel: w438 -> [w523]
        tunnel: [w522] -> w436
        tunnel: w440 -> [w532]
        tunnel: [w531] -> w439
        tunnel: w436 -> [w529]
        tunnel: [w528] -> w435
        tunnel: w439 -> [w545]
        tunnel: [w544] -> w432
        tunnel: [w543] -> w430
        tunnel: w435 -> [w543]
        tunnel: w432 -> [w563]
        tunnel: [w563] -> w431
        tunnel: w430 -> [w562]
        tunnel: [w562] -> w429
        tunnel: [w565] -> w428
        tunnel: w431 -> [w565]
        tunnel: [w564] -> w426
        tunnel: w429 -> [w564]
        tunnel: w428 -> [w579]
        tunnel: [w579] -> w427
        tunnel: w426 -> [_]
        tunnel: [w578] -> w425
        tunnel: w427 -> [w585]
        tunnel: w425 -> [w584]
        frame #0 {
          w451 = TRUE ("Reset Encoder")
          n202 = while {
            stop <- w461 stop-if-true
            # "lift up the can\nthat starts in \nthe bot"
            n203 = Wait (ms)(milliseconds to wait=u32 10) -> ()  [unwired: 1 out]
            n204 = call "Elevator Bang Bang.vi"("Top"=TRUE, "Middle"=FALSE, "Bottom"=FALSE) -> ("in range"=w461:bool)  [unwired: 8 in]
          }
          n205 = local write "Reset Encoder"(TRUE ("Reset Encoder")) -> ()
          n206 = call <vilib>:"WPI_SolenoidRefNum Registry Get.vi"("refnum name"="H Drive Down") -> ("SolenoidDevRef"=w447:T2)  [unwired: 9 in, 1 out]
          n207 = call <vilib>:"WPI_SolenoidRefNum Registry Get.vi"("refnum name"="H Drive Up") -> ("SolenoidDevRef"=w448:T2)  [unwired: 9 in, 1 out]
          n208 = call <vilib>:"WPI_GyroRefNum Registry Get.vi"("refnum name"="Gyro") -> ("GyroDevRef"=w458:T16)  [unwired: 9 in, 1 out]
          n209 = Not(x=w451) -> (.not. x?=w450:bool)
          n210 = call <vilib>:"WPI_GyroReset.vi"("GyroDevRef"=w458) -> ()  [unwired: 9 in, 2 out]
          n211 = call-poly <vilib>:"WPI_SolenoidSet.vi"("Value"=w450, "SolenoidDevRef"=w447) -> ()  [unwired: 8 in, 2 out]
          n212 = call-poly <vilib>:"WPI_SolenoidSet.vi"("Value"=w451, "SolenoidDevRef"=w448) -> ()  [unwired: 8 in, 2 out]
          n213 = call "Auto Intake-Elevator-Cangrip.vi"("Intake Wheels (+ is in)"=0.0, "Spin Can"=enum16{"Spin Left", "Spin Right", "Nothing"}."Nothing", "Cangrip Open"=FALSE, "Elevator Open"=FALSE, "Intake Open"=FALSE, "Cluster"=w452) -> ("Output Cluster"=w444:T14)  [unwired: 5 in]
        }
        frame #1 {
          # "23.5"
          # "first turn angle"
          # "turn to point towards\nthe landfill"
          n214 = local write "Reset Encoder"(FALSE ("Reset Encoder")) -> ()
          n215 = call "PID Turn.vi"("Setpoint"=25.0) -> ()  [unwired: 10 in, 1 out]
          n216 = call "Elevator Bang Bang.vi"("Top"=TRUE, "Middle"=FALSE, "Bottom"=FALSE) -> ()  [unwired: 8 in, 1 out]
        }
        frame #2 {
          n217 = flat-sequence {
            tunnel: [w486] -> w475
            tunnel: w475 -> [w488]
            tunnel: [w488] -> w474
            tunnel: w474 -> [w493]
            frame #0 {
              w486 = 4.0 ("Setpoint Distance")
              # "9.2"
              # "first move speed"
              # "first move distance"
              # "drive forward while pulling in\nthe first tote from the landfill"
              n218 = call "Driving Encoder Distance.vi"("Speed"=0.5 ("Setpoint Distance"), "Setpoint Distance"=w486) -> ()  [unwired: 7 in, 3 out]
            }
            frame #1 {
              # "turn into the tote"
              # "reset the gyro"
              n219 = call "PID Turn.vi"("Reset gyro"=TRUE, "Setpoint"=15.0) -> ()  [unwired: 9 in, 1 out]
            }
            frame #2 {
              # "backup  a bit"
              n220 = Subtract(x=w493, y=0.75 ("Setpoint Distance")) -> (x-y=w491:dbl)
              n221 = call "Driving Encoder Distance.vi"("Speed"=-0.5, "Setpoint Distance"=w491) -> ()  [unwired: 7 in, 3 out]
            }
          }
          n222 = call "Elevator Bang Bang.vi"("Top"=TRUE, "Middle"=FALSE, "Bottom"=FALSE) -> ()  [unwired: 8 in, 1 out]
          n223 = call "Auto Intake-Elevator-Cangrip.vi"("Intake Wheels (+ is in)"=1.0, "Spin Can"=enum16{"Spin Left", "Spin Right", "Nothing"}."Nothing", "Cangrip Open"=FALSE, "Elevator Open"=FALSE, "Intake Open"=FALSE, "Cluster"=w477) -> ("Output Cluster"=w476:T14)  [unwired: 5 in]
          n224 = while {
            stop <- w484 stop-if-true
            # "wait for bump switches"
            n225 = call "Check tote in intake.vi"() -> ("Either"=w483:bool)  [unwired: 8 in, 3 out]
            n226 = call "Boolean Delay.vi"("Delay (ms)"=100.0, "Input"=w483) -> ("Output"=w484:bool)  [unwired: 9 in]
          }
        }
        frame #3 {
          # "stop, reset encoders\nand lower elevator"
          n227 = while {
            stop <- w509 stop-if-true
            n228 = Wait (ms)(milliseconds to wait=u32 10) -> ()  [unwired: 1 out]
            n229 = call "Elevator Bang Bang.vi"("Top"=FALSE, "Middle"=FALSE, "Bottom"=TRUE) -> ("in range"=w509:bool)  [unwired: 8 in]
          }
          n230 = local write "Reset Encoder"(TRUE ("Reset Encoder")) -> ()
          n231 = Wait (ms)(milliseconds to wait=u32 250) -> ()  [unwired: 1 out]
          n232 = call <vilib>:"WPI_RobotDriveRefNum Registry Get.vi"("refnum name"="Drive Motors") -> ("RobotDriveDevRef"=w498:T13)  [unwired: 1 in, 9 out]
          n233 = call "Auto Intake-Elevator-Cangrip.vi"("Intake Wheels (+ is in)"=0.0, "Spin Can"=enum16{"Spin Left", "Spin Right", "Nothing"}."Nothing", "Cangrip Open"=FALSE, "Elevator Open"=FALSE, "Intake Open"=FALSE, "Cluster"=w495) -> ("Output Cluster"=w502:T14)  [unwired: 5 in]
          n234 = call <vilib>:"WPI_RobotDriveTankDrive.vi"("Right axis value"=0.0, "Left axis value"=0.0, "RobotDriveDevRef"=w498) -> ()  [unwired: 6 in, 3 out]
        }
        frame #4 {
          n235 = Wait (ms)(milliseconds to wait=u32 260) -> ()  [unwired: 1 out]
        }
        frame #5 {
          # "raise elevator"
          n236 = call "Elevator Bang Bang.vi"("Top"=TRUE, "Middle"=FALSE, "Bottom"=FALSE) -> ()  [unwired: 8 in, 1 out]
        }
        frame #6 {
          # "raise elevator"
          # "-16.5"
          # "turn to face\nthe next tote"
          n237 = call "PID Turn.vi"("Setpoint"=-25.0) -> ("Angel out"=w522:dbl)  [unwired: 10 in]
          n238 = call "Elevator Bang Bang.vi"("Top"=TRUE, "Middle"=FALSE, "Bottom"=FALSE) -> ()  [unwired: 8 in, 1 out]
        }
        frame #7 {
          # "raise elevator"
          # "second move distance"
          # "drive forward while pulling in\nthe second tote from the landfill"
          n239 = while {
            stop <- w541 stop-if-true
            # "wait for bump switches"
            n240 = call "Check tote in intake.vi"() -> ("Either"=w540:bool)  [unwired: 8 in, 3 out]
            n241 = call "Boolean Delay.vi"("Delay (ms)"=250.0, "Input"=w540) -> ("Output"=w541:bool)  [unwired: 9 in]
          }
          n242 = call "Elevator Bang Bang.vi"("Top"=TRUE, "Middle"=FALSE, "Bottom"=FALSE) -> ()  [unwired: 8 in, 1 out]
          n243 = local write "Reset Encoder"(FALSE ("Reset Encoder")) -> ()
          n244 = call "Driving Encoder Distance.vi"("Speed"=0.5 ("Setpoint Distance"), "Setpoint Angle"=w529, "Setpoint Distance"=1.25) -> ("Gyro Angle"=w528:dbl)  [unwired: 6 in, 2 out]
          n245 = call "Auto Intake-Elevator-Cangrip.vi"("Intake Wheels (+ is in)"=1.0, "Spin Can"=enum16{"Spin Left", "Spin Right", "Nothing"}."Nothing", "Cangrip Open"=FALSE, "Elevator Open"=FALSE, "Intake Open"=FALSE, "Cluster"=w532) -> ("Output Cluster"=w531:T14)  [unwired: 5 in]
        }
        frame #8 {
          # "stop, reset encoders\nand lower elevator"
          n246 = while {
            stop <- w557 stop-if-true
            n247 = Wait (ms)(milliseconds to wait=u32 10) -> ()  [unwired: 1 out]
            n248 = call "Elevator Bang Bang.vi"("Top"=FALSE, "Middle"=FALSE, "Bottom"=TRUE) -> ("in range"=w557:bool)  [unwired: 8 in]
          }
          n249 = call <vilib>:"WPI_RobotDriveRefNum Registry Get.vi"("refnum name"="Drive Motors") -> ("RobotDriveDevRef"=w553:T13)  [unwired: 1 in, 9 out]
          n250 = local write "Reset Encoder"(TRUE ("Reset Encoder")) -> ()
          n251 = call "Auto Intake-Elevator-Cangrip.vi"("Intake Wheels (+ is in)"=0.0, "Spin Can"=enum16{"Spin Left", "Spin Right", "Nothing"}."Nothing", "Cangrip Open"=FALSE, "Elevator Open"=FALSE, "Intake Open"=FALSE, "Cluster"=w545) -> ("Output Cluster"=w544:T14)  [unwired: 5 in]
          n252 = call <vilib>:"WPI_RobotDriveTankDrive.vi"("Right axis value"=0.0, "Left axis value"=0.0, "RobotDriveDevRef"=w553) -> ()  [unwired: 6 in, 3 out]
        }
        frame #9 {
          n253 = Wait (ms)(milliseconds to wait=u32 260) -> ()  [unwired: 1 out]
        }
        frame #10 {
          n254 = while {
            stop <- w567 stop-if-true
            # "raise elevator"
            n255 = call "Elevator Bang Bang.vi"("Top"=TRUE, "Middle"=FALSE, "Bottom"=FALSE) -> ("in range"=w567:bool)  [unwired: 8 in]
            n256 = Wait (ms)(milliseconds to wait=u32 10) -> ()  [unwired: 1 out]
          }
          n257 = local write "Reset Encoder"(FALSE ("Reset Encoder")) -> ()
        }
        frame #11 {
          # "raise elevator"
          n258 = local write "Reset Encoder"(TRUE ("Reset Encoder")) -> ()
          n259 = call "Elevator Bang Bang.vi"("Top"=TRUE, "Middle"=FALSE, "Bottom"=FALSE) -> ()  [unwired: 8 in, 1 out]
          n260 = call "PID Turn.vi"("Reset gyro"=TRUE, "Setpoint"=-7.0) -> ("Angel out"=w578:dbl)  [unwired: 9 in]
        }
        frame #12 {
          # "raise elevator"
          # "back away 1 ft"
          n261 = local write "Reset Encoder"(FALSE ("Reset Encoder")) -> ()
          n262 = call "Elevator Bang Bang.vi"("Top"=TRUE, "Middle"=FALSE, "Bottom"=FALSE) -> ()  [unwired: 8 in, 1 out]
          n263 = call "Driving Encoder Distance.vi"("Speed"=-0.5 ("Setpoint Distance"), "Setpoint Angle"=w584, "Setpoint Distance"=-3.5) -> ()  [unwired: 6 in, 3 out]
          n264 = call "Auto Intake-Elevator-Cangrip.vi"("Intake Wheels (+ is in)"=0.0, "Spin Can"=enum16{"Spin Left", "Spin Right", "Nothing"}."Nothing", "Cangrip Open"=FALSE, "Elevator Open"=FALSE, "Intake Open"=FALSE, "Cluster"=w585) -> ()  [unwired: 5 in, 1 out]
        }
        frame #13 {
        }
        frame #14 {
          # "stop. Don't pick up the 3rd tote\nso it's not stressing the elevator"
          n265 = local write "Reset Encoder"(TRUE ("Reset Encoder")) -> ()
          n266 = call <vilib>:"WPI_RobotDriveRefNum Registry Get.vi"("refnum name"="Drive Motors") -> ("RobotDriveDevRef"=w596:T13)  [unwired: 1 in, 9 out]
          n267 = call <vilib>:"WPI_RobotDriveTankDrive.vi"("Right axis value"=0.0, "Left axis value"=0.0, "RobotDriveDevRef"=w596) -> ()  [unwired: 6 in, 3 out]
        }
      }
    }
    frame 6 {
      n268 = flat-sequence {
        tunnel: w598 -> [w599]
        frame #0 {
          w608 = TRUE ("Reset Encoder")
          n269 = call <vilib>:"WPI_SolenoidRefNum Registry Get.vi"("refnum name"="H Drive Down") -> ("SolenoidDevRef"=w604:T2)  [unwired: 9 in, 1 out]
          n270 = call <vilib>:"WPI_SolenoidRefNum Registry Get.vi"("refnum name"="H Drive Up") -> ("SolenoidDevRef"=w605:T2)  [unwired: 9 in, 1 out]
          n271 = Not(x=w608) -> (.not. x?=w607:bool)
          n272 = call <vilib>:"WPI_GyroRefNum Registry Get.vi"("refnum name"="Gyro") -> ("GyroDevRef"=w601:T16)  [unwired: 9 in, 1 out]
          n273 = call-poly <vilib>:"WPI_SolenoidSet.vi"("Value"=w607, "SolenoidDevRef"=w604) -> ()  [unwired: 8 in, 2 out]
          n274 = call-poly <vilib>:"WPI_SolenoidSet.vi"("Value"=w608, "SolenoidDevRef"=w605) -> ()  [unwired: 8 in, 2 out]
          n275 = call <vilib>:"WPI_GyroReset.vi"("GyroDevRef"=w601) -> ()  [unwired: 9 in, 2 out]
          n276 = call "Auto Intake-Elevator-Cangrip.vi"("Intake Wheels (+ is in)"=0.0, "Spin Can"=enum16{"Spin Left", "Spin Right", "Nothing"}."Nothing", "Cangrip Open"=FALSE, "Elevator Open"=FALSE, "Intake Open"=FALSE, "Cluster"=w599) -> ()  [unwired: 5 in, 1 out]
        }
        frame #1 {
          # "first turn angle"
          n277 = call "PID Turn.vi"("Setpoint"=45.0) -> ()  [unwired: 10 in, 1 out]
        }
      }
    }
  }
  n278 = call <vilib>:"WPI_PotentiometerRefNum Registry Get.vi"("refnum name"="Pot") -> ("PotDevRef"=w8:T19)  [unwired: 9 in, 1 out]
  n279 = call <vilib>:"WPI_EncoderRefNum Registry Get.vi"("refnum name"="Drive Encoder Left") -> ("EncoderDevRef"=w40:T20)  [unwired: 9 in, 1 out]
  n280 = call <vilib>:"WPI_EncoderRefNum Registry Get.vi"("refnum name"="Drive Encoder Right") -> ("EncoderDevRef"=w39:T20)  [unwired: 9 in, 1 out]
  n281 = call <vilib>:"WPI_GyroRefNum Registry Get.vi"("refnum name"="Gyro") -> ("GyroDevRef"=w6:T16)  [unwired: 9 in, 1 out]
  n282 = while {
    tunnel: w40 -> [w632]
    tunnel: w39 -> [w629]
    tunnel: w8 -> [w619]
    tunnel: w6 -> [w618]
    stop <- FALSE stop-if-true
    n283 = call <vilib>:"WPI_GyroGetAngle.vi"("GyroDevRef"=w618) -> ("Angle"=w617:dbl)  [unwired: 7 in, 3 out]
    n284 = call <vilib>:"WPI_PotentiometerGetNormalized.vi"("PotDevRef"=w619) -> ("Normalized Value"=w621:dbl)  [unwired: 8 in, 2 out]
    "Pot Value" <- w621
    n285 = case shown="False" "Reset Encoder" {
      tunnel: w632 -> [w635 w640]
      tunnel: [w635 w639] -> w631
      tunnel: w629 -> [w636 w637]
      tunnel: [w636 w638] -> w630
      frame False {
      }
      frame True {
        n286 = call <vilib>:"WPI_EncoderReset.vi"("EncoderDevRef"=w640) -> ("EncoderDevRef"=w639:T20)  [unwired: 9 in, 1 out]
        n287 = call <vilib>:"WPI_EncoderReset.vi"("EncoderDevRef"=w637) -> ("EncoderDevRef"=w638:T20)  [unwired: 9 in, 1 out]
      }
    }
    n288 = call-poly <vilib>:"SD Write Value.vi"("Numeric"=w617, "Name"="Gyro") -> ()  [unwired: 8 in, 2 out]
    n289 = call-poly <vilib>:"SD Write Value.vi"("Numeric"=w621, "Name"="Pot Value") -> ()  [unwired: 8 in, 2 out]
    n290 = call <vilib>:"WPI_EncoderGet.vi"("EncoderDevRef"=w631) -> ("Distance"=w624:dbl)  [unwired: 5 in, 5 out]
    n291 = call <vilib>:"WPI_EncoderGet.vi"("EncoderDevRef"=w630) -> ("Distance"=w625:dbl)  [unwired: 5 in, 5 out]
    n292 = Absolute Value(x=w624) -> (abs(x)=w623:dbl)
    "L Encoder" <- w623
    n293 = Absolute Value(x=w625) -> (abs(x)=w622:dbl)
    "R Encoder" <- w622
    n294 = Add(x=w623, y=w622) -> (x+y=w628:dbl)
    n295 = Divide(x=w628, y=2.0) -> (x/y=w614:dbl)
    "Avg Encoder" <- w614
    n296 = call-poly <vilib>:"SD Write Value.vi"("Numeric"=w614, "Name"="Encoder") -> ()  [unwired: 8 in, 2 out]
    n297 = Wait (ms)(milliseconds to wait=u32 10) -> ()  [unwired: 1 out]
  }
